vi "Empty Data Check(SIM).vi"(11 "Cluster Data":T1) -> (3 "Empty?":bool)   [LabVIEW 2021]
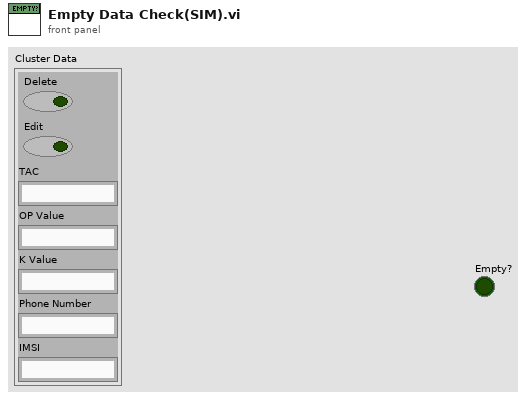
[diagram p1: front panel]
types:
  T1 = cluster{"Delete":bool, "Edit":bool, "TAC":string, "OP Value":string, "K Value":string, "Phone Number":string, "IMSI":string}
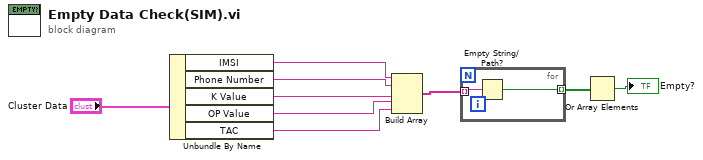
[diagram p0: block diagram]
diagram:
  n1 = Unbundle By Name("Cluster Data") -> ("IMSI"=w5:string, "Phone Number"=w6:string, "K Value"=w7:string, "OP Value"=w8:string, "TAC"=w9:string)
  n2 = Build Array(w5, w6, w7, w8, w9) -> (w4:string[])
  n3 = for {
    tunnel: w4 -> [w11] mode=indexing
    tunnel: [w10] -> w3 mode=indexing
    n4 = Empty String/Path?(string/path=w11) -> (empty?=w10:bool)
  }
  n5 = Or Array Elements(Boolean array=w3) -> (logical OR=→"Empty?":bool)
